vi "ParamMaster.vi"() -> ()   [LabVIEW 2014]
panel:
  out "Warning":bool
  out "Message":string
  out "Cat to name ?":bool[](array[boolean])
  in  "Parameters and values":string[][](array[string])
  in  "Stop Button":bool
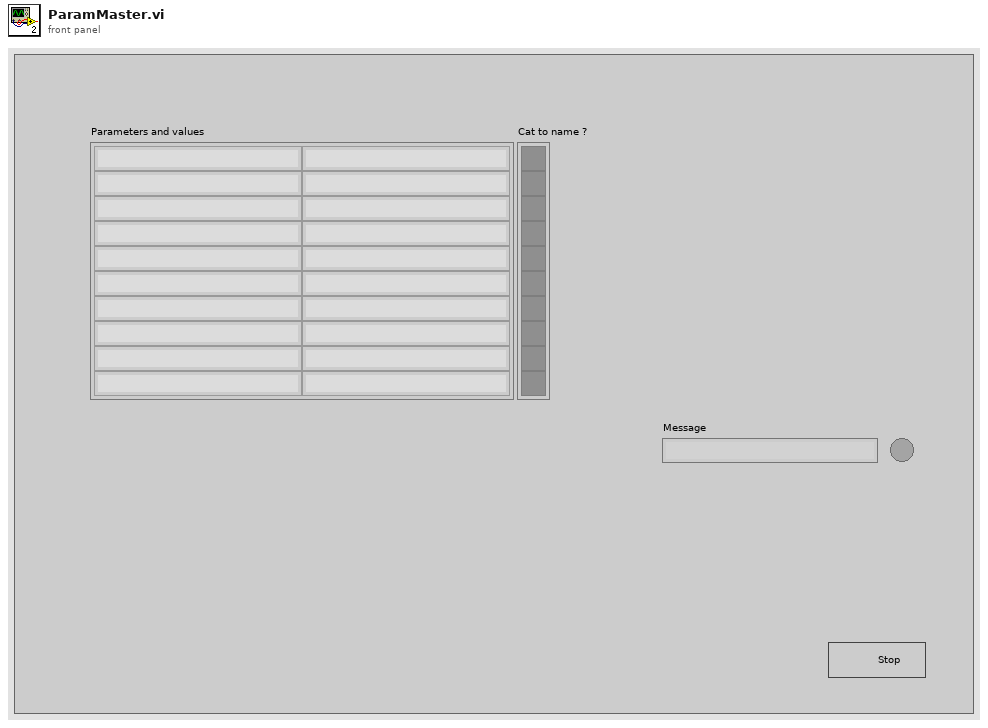
[diagram p1: front panel]
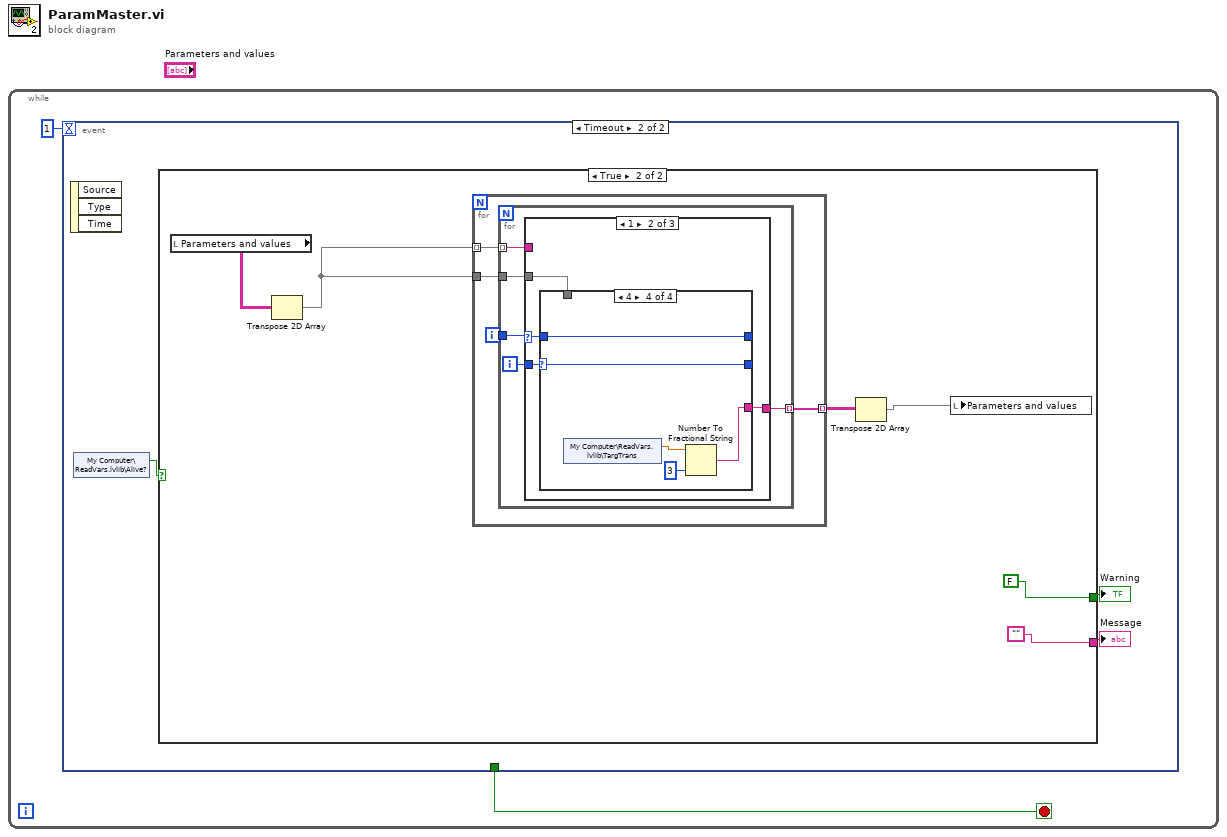
[diagram p0: block diagram]
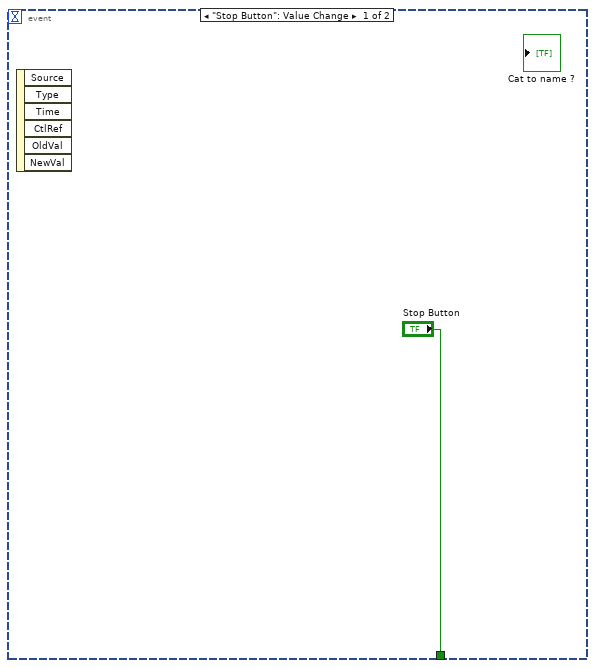
[diagram p2: hidden frame]
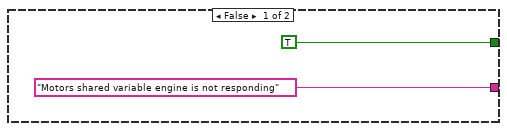
[diagram p3: hidden frame]
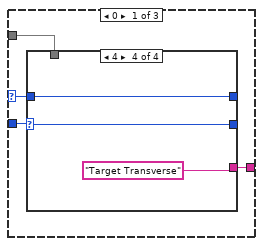
[diagram p4: hidden frame]
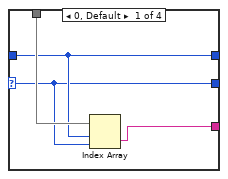
[diagram p5: hidden frame]
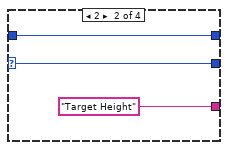
[diagram p6: hidden frame]
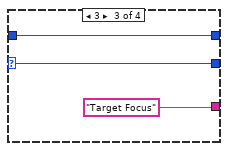
[diagram p7: hidden frame]
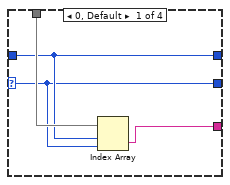
[diagram p8: hidden frame]
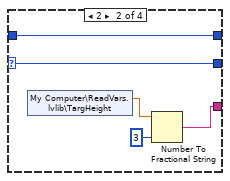
[diagram p9: hidden frame]
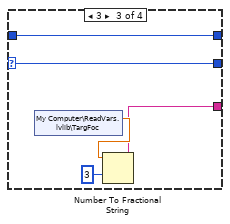
[diagram p10: hidden frame]
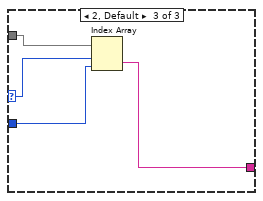
[diagram p11: hidden frame]
diagram:
  n1 = while {
    stop <- w2 stop-if-true
    n2 = event shown="[1] Timeout" {
      selector: _ -> [_ _]
      dyn-events: _ -> [_ _]
      timeout: 1 -> [_ _]
      tunnel: ["Stop Button" _] -> w2
      event "Stop Button": Value Change {
        n3 = event-data() -> ()  [unwired: 1 in, 6 out]
      }
      event Timeout {
        n4 = event-data() -> ()  [unwired: 1 in, 3 out]
        n5 = shared-variable "My Computer\\ReadVars.lvlib\\Alive?"() -> (w6:bool)  [unwired: 1 in, 1 out]
        n6 = case shown="True" w6 {
          tunnel: ["Motors shared variable engine is not responding" ""] -> w5
          tunnel: [TRUE FALSE] -> w4
          frame False {
          }
          frame True {
            n7 = local read "Parameters and values"() -> (w12:string[][])
            n8 = Transpose 2D Array(2D array=w12) -> (transposed array=w11:string[][])
            n9 = for {
              tunnel: w11 -> [w18] mode=indexing
              tunnel: w11 -> [w16]
              tunnel: [w15] -> w10 mode=indexing
              i -> [w17]
              n10 = for {
                tunnel: w18 -> [w22] mode=indexing
                tunnel: w17 -> [w23]
                tunnel: w16 -> [w21]
                tunnel: [w19] -> w15 mode=indexing
                i -> [w20]
                n11 = case shown="1" w23 {
                  selector: w23 -> [w26 w44 w66]
                  tunnel: w22 -> [_ _ _]
                  tunnel: w21 -> [w24 w41 w67]
                  tunnel: w20 -> [w27 w43 w65]
                  tunnel: [w25 w42 w64] -> w19
                  frame 0 {
                    n12 = case shown="4" w27 {
                      selector: w27 -> [w29 w33 w35 w38]
                      tunnel: [w30 w34 w36 w39] -> _
                      tunnel: w26 -> [w30 w34 w36 w39]
                      tunnel: [w29 w33 w35 w38] -> _
                      tunnel: [w28 "Target Height" "Target Focus" "Target Transverse"] -> w25
                      tunnel: w24 -> [w31 _ _ _]
                      frame 0, Default {
                        n13 = Index Array(array=w31, index (row)=w30, index (col)=w29) -> (element=w28:string)
                      }
                      frame 2 {
                      }
                      frame 3 {
                      }
                      frame 4 {
                      }
                    }
                  }
                  frame 1 {
                    n14 = case shown="4" w43 {
                      selector: w43 -> [w46 w52 w56 w60]
                      tunnel: [w47 w53 w55 w61] -> _
                      tunnel: w44 -> [w47 w53 w55 w61]
                      tunnel: [w46 w52 w56 w60] -> _
                      tunnel: [w45 w50 w57 w62] -> w42
                      tunnel: w41 -> [w48 _ _ _]
                      frame 0, Default {
                        n15 = Index Array(array=w48, index (row)=w47, index (col)=w46) -> (element=w45:string)
                      }
                      frame 2 {
                        n16 = shared-variable "My Computer\\ReadVars.lvlib\\TargHeight"() -> (w51:dbl)  [unwired: 1 in, 1 out]
                        n17 = Number To Fractional String(number=w51, precision (6)=i16 3) -> (F-format string=w50:string)  [unwired: 2 in]
                      }
                      frame 3 {
                        n18 = shared-variable "My Computer\\ReadVars.lvlib\\TargFoc"() -> (w58:dbl)  [unwired: 1 in, 1 out]
                        n19 = Number To Fractional String(number=w58, precision (6)=i16 3) -> (F-format string=w57:string)  [unwired: 2 in]
                      }
                      frame 4 {
                        n20 = shared-variable "My Computer\\ReadVars.lvlib\\TargTrans"() -> (w63:dbl)  [unwired: 1 in, 1 out]
                        n21 = Number To Fractional String(number=w63, precision (6)=i16 3) -> (F-format string=w62:string)  [unwired: 2 in]
                      }
                    }
                  }
                  frame 2, Default {
                    n22 = Index Array(array=w67, index (row)=w66, index (col)=w65) -> (element=w64:string)
                  }
                }
              }
            }
            n23 = Transpose 2D Array(2D array=w10) -> (transposed array=w9:string[][])
            n24 = local write "Parameters and values"(w9) -> ()
          }
        }
        "Warning" <- w4
        "Message" <- w5
      }
    }
  }
